vi "NetworkTriggerDAQ.vi"() -> ()   [LabVIEW 2020]
uses:
  <vilib>/addons/zeromq/socket_type.ctl
  <vilib>/DAQmx/read.llb/DAQmx Read (Analog Wfm 1Chan NSamp).vi
  <vilib>/DAQmx/miscellaneous.llb/DAQmx Fill In Error Info.vi
  <vilib>/addons/zeromq/zmq_context.lvclass
  <vilib>/addons/zeromq/zmq_socket.lvclass
  <vilib>/addons/zeromq/zeromq.lvlib
panel:
  out "time string":string
  in  "endpoint":string="tcp://192.168.14.15:" caption="endpoint (publisher IP)"
  in  "port":i32=5555
  out "data":waveform(dbl)
  out "Numeric":i32
  out "error out":errorcluster
  in  "stop":bool
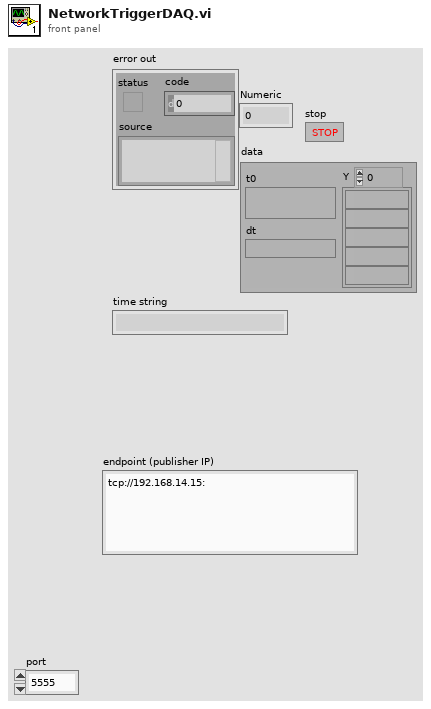
[diagram p1: front panel]
types:
  T1 = typedef "zeromq.lvlib/socket_type.ctl" = enum8{"ZMQ_PAIR", "ZMQ_PUB", "ZMQ_SUB", "ZMQ_REQ", "ZMQ_REP", "ZMQ_DEALER", "ZMQ_ROUTER", "ZMQ_PULL", "ZMQ_PUSH", "ZMQ_XPUB", "ZMQ_XSUB", "ZMQ_STREAM", "ZMQ_SERVER", "ZMQ_CLIENT", "ZMQ_RADIO", "ZMQ_DISH", "ZMQ_GATHER", "ZMQ_SCATTER", "ZMQ_DGRAM"}
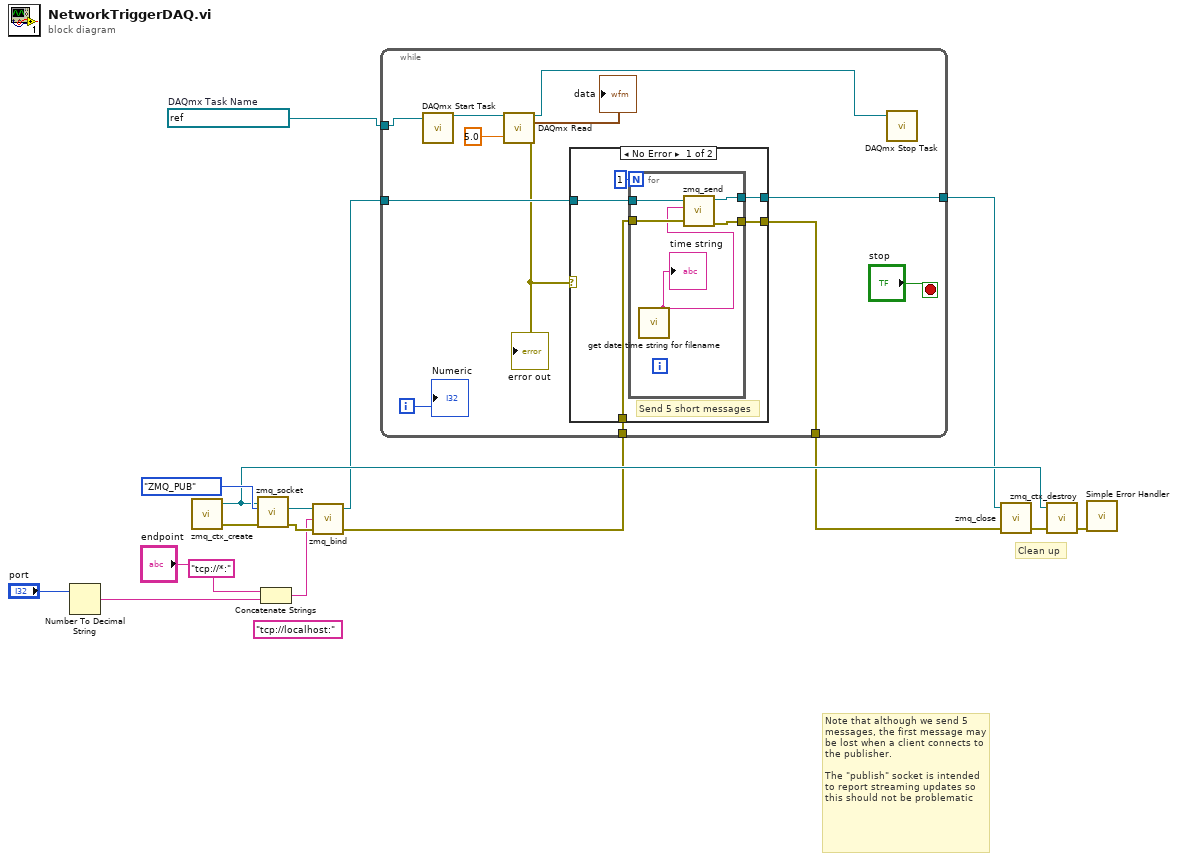
[diagram p0: block diagram]
diagram:
  (unwired) "tcp://localhost:" ("endpoint")
  (unwired) "tcp://*:" ("endpoint")
  w16 = refnum<k21> "AcquireOnTrigger"  # DAQmx Task Name
  # "Note that although we send 5 messages, the first message may be lost when a client connects to the publisher.\n\nThe \"publish\" socket is intended to report streaming updates so this should not be problematic"
  # "Clean up"
  n1 = Number To Decimal String(number="port") -> (decimal integer string=w7:string)  [unwired: 1 in]
  n2 = call <vilib>:"zmq_ctx_create.vi"() -> ("error out"=w14:errorcluster, "context out"=w10:refnum<class "zmq_context.lvclass">)  [unwired: 4 in]
  n3 = call <vilib>:"zmq_socket.vi"("error in"=w14, "socket type"=socket_type."ZMQ_PUB", "context in"=w10) -> ("error out"=w13:errorcluster, "socket out"=w9:refnum<class "zmq_socket.lvclass">)  [unwired: 2 in, 1 out]
  n4 = Concatenate Strings("endpoint", w7) -> (w6:string)
  n5 = call <vilib>:"zmq_bind.vi"("error in"=w13, "endpoint"=w6, "socket in"=w9) -> ("error out"=w3:errorcluster, "socket out"=w4:refnum<class "zmq_socket.lvclass">)  [unwired: 1 in]
  n6 = while {
    tunnel: w16 -> [w24]
    tunnel: w4 -> [w21]
    tunnel: w3 -> [w20]
    tunnel: [w19] -> w2
    tunnel: [w18] -> w1
    i -> [w26]
    stop <- "stop" stop-if-true
    n7 = call <vilib>:"DAQmx Start Task.vi"("task/channels in"=w24) -> ("task out"=w23:refnum<k21>)  [unwired: 13 in, 1 out]
    n8 = call-poly <vilib>:"DAQmx Read.vi"("task/channels in"=w23, "timeout"=5.0) -> ("task out"=w22:refnum<k21>, "data"=→"data":waveform(dbl), "error out"=w17:errorcluster)  [unwired: 11 in]
    "error out" <- w17
    n9 = case shown="No Error" w17 {
      tunnel: w21 -> [w32 w40]
      tunnel: w20 -> [w31 w39]
      tunnel: [w30 w40] -> w19
      tunnel: [w29 w39] -> w18
      frame No Error {
        # "Send 5 short messages"
        n10 = for {
          N: 1 -> [_]
          tunnel: w32 -> [w38]
          tunnel: w31 -> [w37]
          tunnel: [w36] -> w30
          tunnel: [w35] -> w29
          n11 = call "get date time string for filename.vi"() -> ("time string"=w34:string)  [unwired: 11 in]
          "time string" <- w34
          n12 = call <vilib>:"zmq_send.vi"("error in"=w37, "data"=w34, "socket in"=w38) -> ("error out"=w35:errorcluster, "socket out"=w36:refnum<class "zmq_socket.lvclass">)  [unwired: 4 in]
        }
      }
      frame Error {
      }
    }
    n13 = call <vilib>:"DAQmx Stop Task.vi"("task/channels in"=w22) -> ()  [unwired: 13 in, 2 out]
    "Numeric" <- w26
  }
  n14 = call <vilib>:"zmq_close.vi"("error in"=w1, "socket"=w2) -> ("error out"=w11:errorcluster)  [unwired: 3 in]
  n15 = call <vilib>:"zmq_ctx_destroy.vi"("error in"=w11, "context in"=w10) -> ("error out"=w12:errorcluster)  [unwired: 3 in]
  n16 = call <vilib>:"Simple Error Handler.vi"("error in (no error)"=w12) -> ()  [unwired: 4 in, 5 out]
